vi "Calibrate Potentiometer.vi"(7 "Unit Address (1)":u8=1, 8 "error in (no error)":errorcluster, 10 "Calibrate Potentiometer (False)":bool, 11 "VISA resource name":refnum<visa-resource-name>) -> (0 "error out":errorcluster, 3 "VISA resource name out":refnum<visa-resource-name>)   [LabVIEW 2014, in "Eurotherm 35xx Series.lvlib"]
doc: "This VI starts the potentiometer calibration by selecting which valves potentiometer to calibrate. e.g. if a valve is used to control the cooling of a process, then the ch2 potentiometer must be calibrated.\n\nNote: Potentiometer input modules must be fitted and wired directly to the loops Ch1 or Ch2 pot position parameters."
uses:
  <instrlib>/Eurotherm 35xx Series/Eurotherm 35xx Series.lvlib
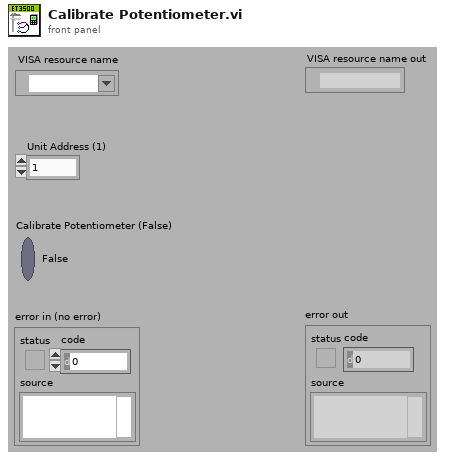
[diagram p1: front panel]
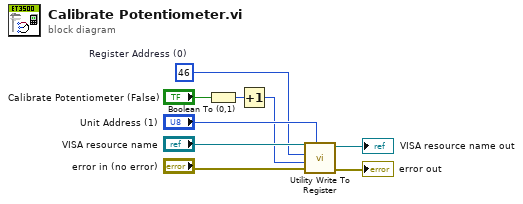
[diagram p0: block diagram]
diagram:
  w4 = 46  # Register Address (0)
  n1 = Boolean To (0,1)(Boolean="Calibrate Potentiometer (False)") -> (0, 1=w2:i16)
  n2 = Increment(x=w2) -> (x+1=w1:i16)
  n3 = call <instrlib>:"Utility Write To Register.vi"("Unit Address (1)"="Unit Address (1)", "error in (no error)"="error in (no error)", "Data (0)"=w1, "Register Address (0)"=w4, "VISA resource name"="VISA resource name") -> ("error out"=→"error out":errorcluster, "VISA resource name out"=→"VISA resource name out":refnum<visa-resource-name>)  [unwired: 5 in]
